vi "Rapidox parse RT.vi"() -> (2 "O2 %":dbl)   [LabVIEW 2011]
uses:
  <vilib>/rvi/interface/nirviOpenFPGA/nirviOpenFPGA.xnode
  <vilib>/rvi/interface/nirviReadWriteControl/nirviReadWriteControl.xnode
  NiFpgaLv.dll
  <vilib>/Utility/error.llb/Error Cluster From Error Code.vi
  <vilib>/rvi/interface/Simulation/niFpgaSimulationCallBeginRW.vi
  <vilib>/rvi/errors/niLvFpgaAdjustHostInterfaceError.vi
  <vilib>/rvi/interface/nirviCloseFPGA/nirviCloseFPGA.xnode
  <vilib>/FPGAPlugInAG/Dynamic/niLvFpga_Close_Dynamic.vi
  FPGA Bitfiles/MAXCATTestProjec_FPGATarget2_RapidoxreadMAXFP_208F814E.lvbitx
  Rapidox read MAX FPGA.vi
  <vilib>/FPGAPlugInAG/cRIO-9074/niLvFpga_Open_cRIO-9074.vi
  <vilib>/rvi/interface/common/dynamic/niFpgaDynamicAddResources.vi
panel:
  in  "stop":bool
  # "rapidox array"
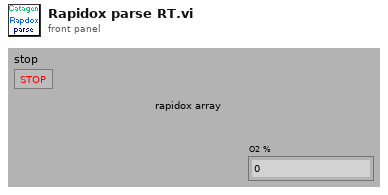
[diagram p1: front panel]
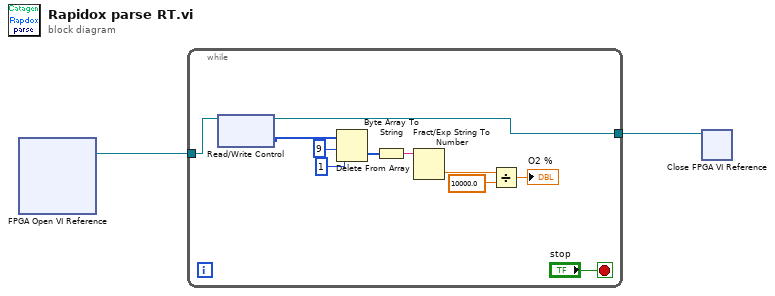
[diagram p0: block diagram]
diagram:
  n1 = xnode "FPGA Open VI Reference"() -> ("FPGA VI Reference Out"=w2:refnum<k20>)  [unwired: 2 in, 1 out]
  n2 = while {
    tunnel: w2 -> [w6]
    tunnel: [w3] -> w1
    stop <- "stop" stop-if-true
    n3 = xnode "Read/Write Control"("FPGA VI Reference In"=w6) -> ("FPGA VI Reference Out"=w3:refnum<k20>, "Output"=w5:u8[])  [unwired: 1 in, 1 out]
    n4 = Delete From Array(array=w5, length=9, index=1) -> (deleted portion=w10:u8[])  [unwired: 1 out]
    n5 = Byte Array To String(unsigned byte array=w10) -> (string=w9:string)
    n6 = Fract/Exp String To Number(string=w9) -> (number=w8:dbl)  [unwired: 3 in, 1 out]
    n7 = Divide(x=w8, y=10000.0) -> (x/y=→"O2 %":dbl)
  }
  n8 = xnode "Close FPGA VI Reference"("FPGA VI Reference In"=w1) -> ()  [unwired: 1 in, 1 out]
